vi "YAML_readtest.vi"(11 "ENTIRE Array of YAML Lines":string[](array[string])) -> ()   [LabVIEW 2016]
panel:
  out "size":i32
  out "items in subdirectory":cluster{"key":variant, "value":variant}[](array[cluster])
  out "value":variant
  out "Dictionary Items":cluster{"key":variant, "value":variant}[](array[cluster])
  out "keys":variant[](array[variant])
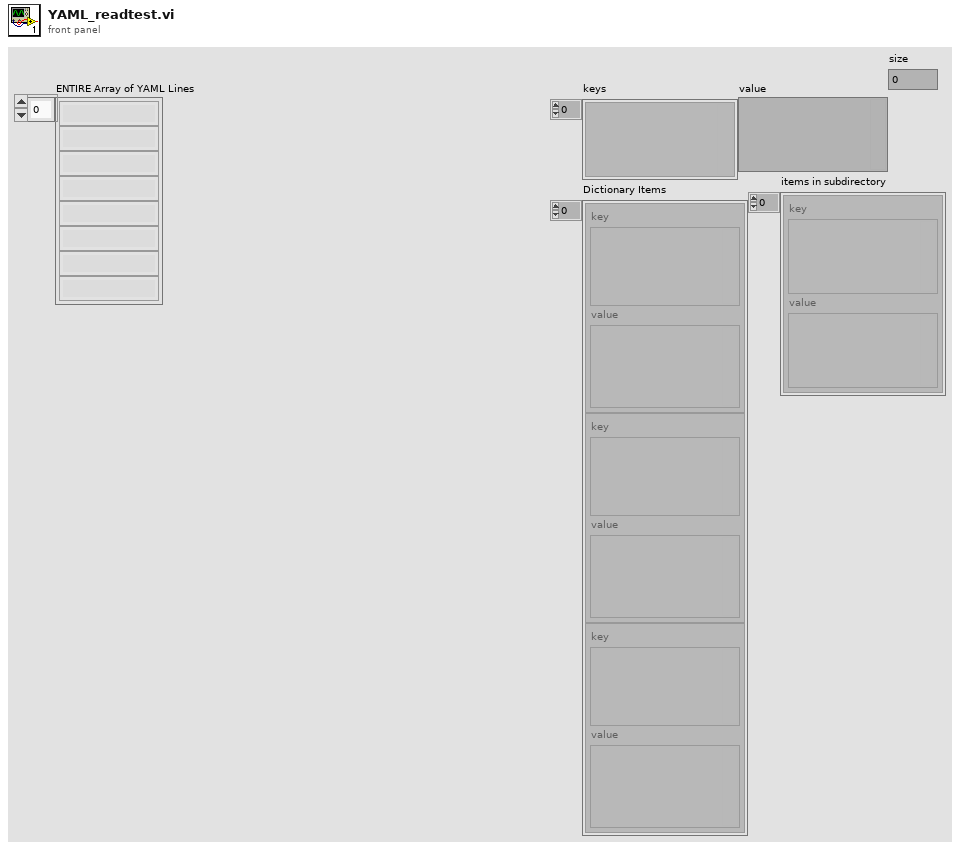
[diagram p1: front panel]
types:
  T1 = typedef "Dictionary Object RefNum__ogtk.ctl" = refnum<k1>
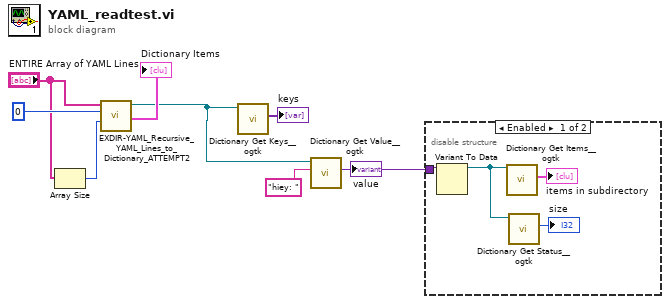
[diagram p0: block diagram]
diagram:
  n1 = Array Size(array="ENTIRE Array of YAML Lines") -> (size(s)=w5:i32)
  n2 = call "EXDIR-YAML_Recursive_YAML_Lines_to_Dictionary_ATTEMPT2.vi"("End Index"=w5, "Start Index"=0, "ENTIRE Array of YAML Lines"="ENTIRE Array of YAML Lines") -> ("items"=→"Dictionary Items":cluster{"key":variant, "value":variant}[], "dictionary out"=w1:T1)  [unwired: 7 in]
  n3 = call <userlib>:"Dictionary Get Keys__ogtk.vi"("dictionary"=w1) -> ("keys"=→"keys":variant[])  [unwired: 8 in, 2 out]
  n4 = call <userlib>:"Dictionary Get Value__ogtk.vi"("key"="hiey: ", "dictionary"=w1) -> ("value"=w3:variant)  [unwired: 6 in, 3 out]
  "value" <- w3
  n5 = disable-structure shown="Enabled" {
    disable-tunnel: w3 -> [w12 _]
    frame Enabled {
      n6 = Variant To Data(Variant=w12) -> (data=w10:T1)  [unwired: 2 in, 1 out]
      n7 = call <userlib>:"Dictionary Get Items__ogtk.vi"("dictionary"=w10) -> ("items"=→"items in subdirectory":cluster{"key":variant, "value":variant}[])  [unwired: 8 in, 2 out]
      n8 = call <userlib>:"Dictionary Get Status__ogtk.vi"("dictionary"=w10) -> ("size"=→"size":i32)  [unwired: 8 in, 2 out]
    }
    frame Disabled {
    }
  }
